vi "Test MQTT-4.8.0-1.vi"(8 "error in (no error)":errorcluster, 11 "Connection Config":refnum<class "Connection.lvclass">) -> (0 "error out":errorcluster, 3 "Connection Config dup":refnum<class "Connection.lvclass">)   [LabVIEW 2013]
uses:
  <vilib>/addons/_JKI Toolkits/Caraya/classes/Test/Test.lvclass
  <vilib>/LabVIEW Open Source Project/MQTT Control Packets/Control Packets/CONNECT/CONNECT.lvclass
  <vilib>/LabVIEW Open Source Project/MQTT Control Packets/Control Packets/ControlPacket/ControlPacket.lvclass
  <vilib>/addons/_JKI Toolkits/Caraya/classes/Assert/Assert.lvclass
  <vilib>/LabVIEW Open Source Project/Connection/Connection/Connection.lvclass
  <vilib>/LabVIEW Open Source Project/MQTT Control Packets/Control Packets/PUBLISH/PUBLISH.lvclass
  <vilib>/LabVIEW Open Source Project/MQTT Connection/MQTT_Connection/Connection/Connection.lvclass
  <vilib>/LabVIEW Open Source Project/MQTT Control Packets/Control Packets/ControlPacket/Control Packet Type -- enum.ctl
panel:
  out "Should not receive Puback":T1
  out "Connack Packet received?":T1
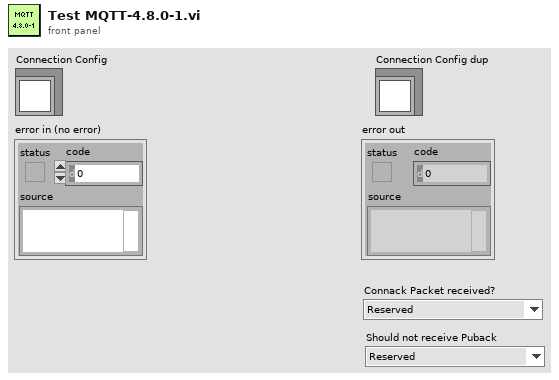
[diagram p1: front panel]
types:
  T1 = typedef "MQTT_Control_Packets.lvlib/ControlPacket.lvclass/Control Packet Type -- enum.ctl" = enum16{"Reserved", "CONNECT", "CONNACK", "PUBLISH", "PUBACK", "PUBREC", "PUBREL", "PUBCOMP", "SUBSCRIBE", "SUBACK", "UNSUBSCRIBE", "UNSUBACK", "PINGREQ", "PINGRESP", "DISCONNECT", "AUTH"}
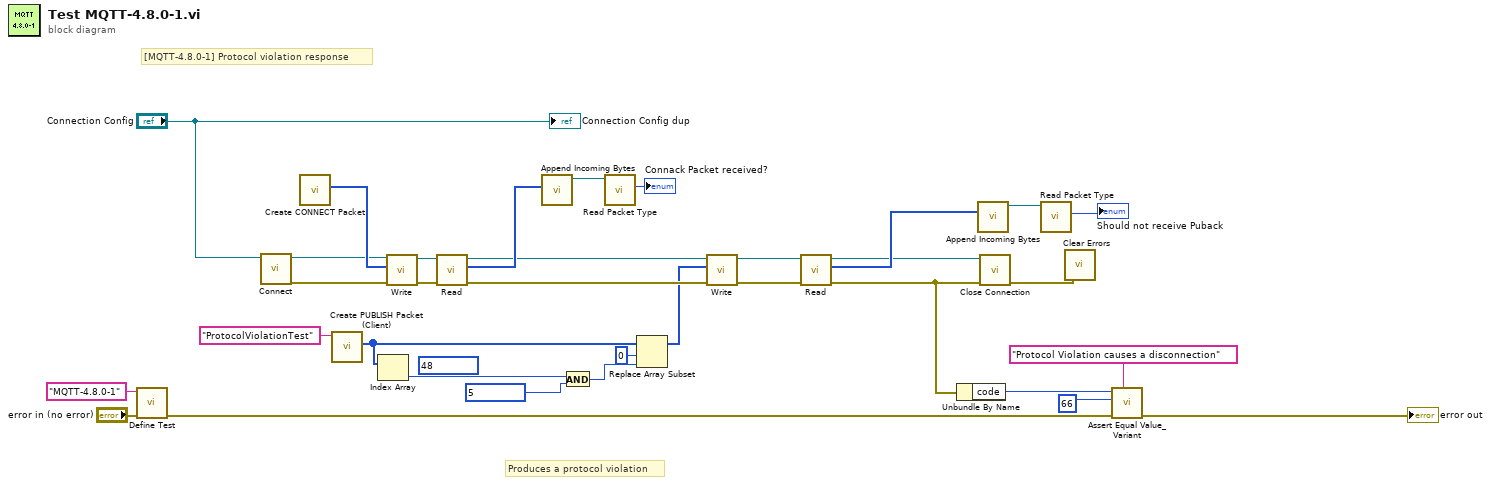
[diagram p0: block diagram]
diagram:
  (unwired) u8 48
  # "Produces a protocol violation"
  # "[MQTT-4.8.0-1] Protocol violation response"
  n1 = call <vilib>:"Define Test.vi"("error in (no error)"="error in (no error)", "Label (VI Title)"="MQTT-4.8.0-1") -> ("error out"=w30:errorcluster)  [unwired: 9 in]
  n2 = call <vilib>:"Connect.vi"("Connection in"="Connection Config") -> ("error out"=w21:errorcluster, "Connection out"=w13:refnum<class "Connection.lvclass">)  [unwired: 9 in]
  n3 = call <vilib>:"Create CONNECT Packet.vi"() -> ("Bytes Stream"=w22:u8[])  [unwired: 9 in, 2 out]
  n4 = call <vilib>:"Create PUBLISH Packet (Client).vi"("Topic Name"="ProtocolViolationTest") -> ("Bytes Stream"=w3:u8[])  [unwired: 7 in, 3 out]
  n5 = Index Array(array=w3) -> (element=w2:u8)  [unwired: 1 in]
  n6 = call <vilib>:"Write.vi"("error in (no error)"=w21, "Bytes"=w22, "Connection in"=w13) -> ("error out"=w20:errorcluster, "Connection"=w19:refnum<class "Connection.lvclass">)  [unwired: 7 in]
  n7 = call <vilib>:"Read.vi"("error in (no error)"=w20, "TCPConnection in"=w19) -> ("error out"=w9:errorcluster, "Bytes"=w18:u8[], "TCPConnection out"=w11:refnum<class "Connection.lvclass">)  [unwired: 5 in, 2 out]
  n8 = call <vilib>:"Append Incoming Bytes.vi"("Incoming Packets"=w18) -> ("ControlPacket"=w29:refnum<class "ControlPacket.lvclass">)  [unwired: 7 in, 3 out]
  n9 = And(x=w2, y=u8 5 ("Byte")) -> (x .and. y?=w1:u8)
  n10 = call <vilib>:"Read Packet Type.vi"("ControlPacket in"=w29) -> ("Control Packet Type"=→"Connack Packet received?":T1)  [unwired: 9 in, 1 out]
  n11 = Replace Array Subset(array=w3, new element=w1, index=0) -> (w6:u8[])
  n12 = call <vilib>:"Write.vi"("error in (no error)"=w9, "Bytes"=w6, "Connection in"=w11) -> ("error out"=w8:errorcluster, "Connection"=w10:refnum<class "Connection.lvclass">)  [unwired: 7 in]
  n13 = call <vilib>:"Read.vi"("error in (no error)"=w8, "TCPConnection in"=w10) -> ("error out"=w15:errorcluster, "Bytes"=w17:u8[], "TCPConnection out"=w16:refnum<class "Connection.lvclass">)  [unwired: 5 in, 2 out]
  n14 = Unbundle By Name(w15) -> ("code"=w25:i32)
  n15 = call <vilib>:"Append Incoming Bytes.vi"("Incoming Packets"=w17) -> ("ControlPacket"=w27:refnum<class "ControlPacket.lvclass">)  [unwired: 7 in, 3 out]
  n16 = call <vilib>:"Close Connection.vi"("error in (no error)"=w15, "Connection in"=w16) -> ("error out"=w14:errorcluster)  [unwired: 8 in, 1 out]
  n17 = call <vilib>:"Read Packet Type.vi"("ControlPacket in"=w27) -> ("Control Packet Type"=→"Should not receive Puback":T1)  [unwired: 9 in, 1 out]
  n18 = call <vilib>:"Clear Errors.vi"("error in (no error)"=w14) -> ()  [unwired: 6 in, 1 out]
  n19 = call <vilib>:"Assert Equal Value_Variant.vi"("Label"="Protocol Violation causes a disconnection", "error in (no error)"=w30, "Y"=66 ("code"), "X"=w25) -> ("error out"=→"error out":errorcluster)  [unwired: 7 in]
  "Connection Config dup" <- "Connection Config"
